vi "configure.vi"(8 "error in (no error)":errorcluster, 11 "RS232 in":refnum<class "RS232.lvclass">) -> (0 "error out":errorcluster, 3 "RS232 out":refnum<class "RS232.lvclass">)   [LabVIEW 2012, in "RS232.lvclass"]
uses:
  RS232.lvclass
  RS232.lvclass/RS232.ctl
  <vilib>/Instr/_visa.llb/VISA Configure Serial Port (Instr).vi
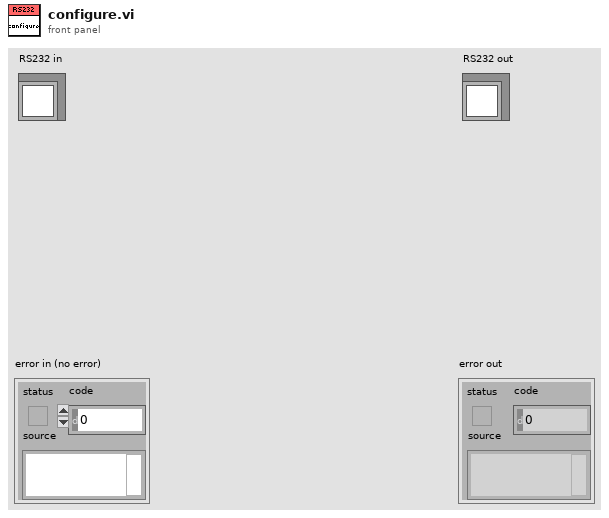
[diagram p1: front panel]
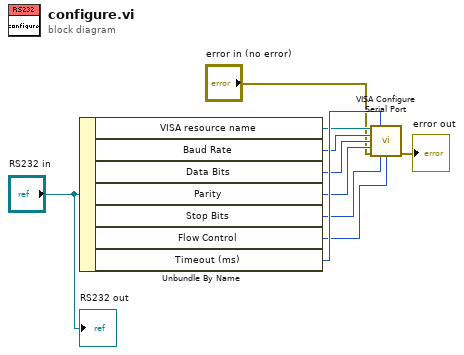
[diagram p0: block diagram]
diagram:
  n1 = Unbundle By Name("RS232 in") -> ("VISA resource name"=w9:refnum<visa-resource-name>, "Baud Rate"=w8:u32, "Data Bits"=w7:u16, "Parity"=w6:enum16{"None", "Odd", "Even", "Mark", "Space"}, "Stop Bits"=w5:u16, "Flow Control"=w4:u16, "Timeout (ms)"=w10:u32)
  n2 = call-poly "VISA Configure Serial Port"("VISA resource name"=w9, "timeout (10sec)"=w10, "baud rate (9600)"=w8, "data bits (8)"=w7, "parity (0:none)"=w6, "error in (no error)"="error in (no error)", "stop bits (10: 1 bit)"=w5, "flow control (0:none)"=w4) -> ("error out"=→"error out":errorcluster)  [unwired: 6 in, 1 out]
  "RS232 out" <- "RS232 in"
